vi "State Lua Garbage Collect.vi"(4 "stepmul (majormul)":i32, 6 "stepsize (minormul)":i32, 8 "pause?":bool, 9 "LUA_GC (LUA_GCCOLLECT)":T1=enum."LUA_GCCOLLECT", 10 "error in (no error)":errorcluster, 11 "Lua in":refnum<class "Lua.lvclass">) -> (1 "result":i32, 2 "error out":errorcluster, 3 "Lua out":refnum<class "Lua.lvclass">)   [LabVIEW 2020, in "Lua for LabVIEW.lvlib" / "Lua.lvclass"]
doc: "Controls the garbage collector.\n\nThis function performs several tasks, according to the value of the parameter what. For options that need extra arguments, they are listed after the option.\n\nLUA_GCCOLLECT: Performs a full garbage-collection cycle.\nLUA_GCSTOP: Stops the garbage collector.\nLUA_GCRESTART: Restarts the garbage collector.\nLUA_GCCOUNT: Returns the current amount of memory (in Kbytes) in use by Lua.\nLUA_GCCOUNTB: Returns the remainder of dividing the current amount of bytes of memory in use by Lua by 1024.\nLUA_GCSTEP (int stepsize): Performs an incremental step of garbage collection, corresponding to the allocation of stepsize Kbytes.\nLUA_GCISRUNNING: Returns a boolean that tells whether the collector is running (i.e., not stopped).\nLUA_GCINC (int pause, int stepmul, stepsize): Changes the collector to incremental mode with the given parameters (see §2.5.1). Returns the previous mode (LUA_GCGEN or LUA_GCINC).\nLUA_GCGEN (int minormul, int majormul): Changes the collector to generational mode with the given parameters (see §2.5.2). Returns the previous mode (LUA_GCGEN or LUA_GCINC).\nFor more details about these options, see collectgarbage."
uses:
  Lua.lvclass
  lib/lua.dll/types/LUA_GC.ctl
  Lua.lvclass/Lua.ctl
  lib/lua.dll/lua.dll.lvlib
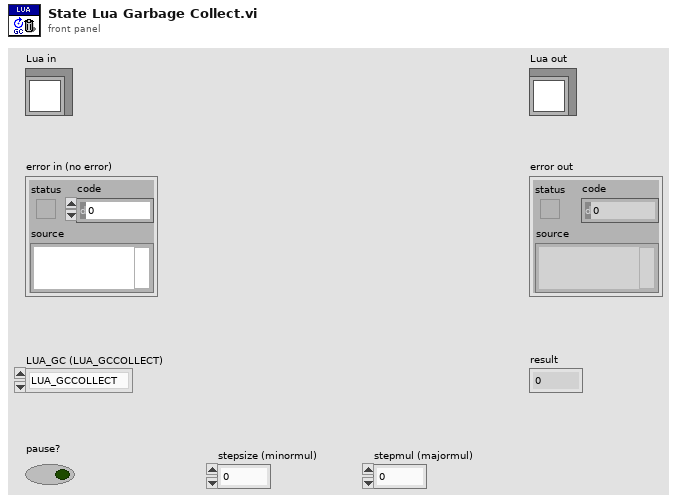
[diagram p1: front panel]
types:
  T1 = typedef "lua.dll.lvlib/LUA_GC.ctl" = enum32{"LUA_GCSTOP", "LUA_GCRESTART", "LUA_GCCOLLECT", "LUA_GCCOUNT", "LUA_GCCOUNTB", "LUA_GCSTEP", "LUA_GCSETPAUSE", "LUA_GCSETSTEPMUL", "LUA_GCSETMAJORINC", "LUA_GCISRUNNING", "LUA_GCGEN", "LUA_GCINC"}
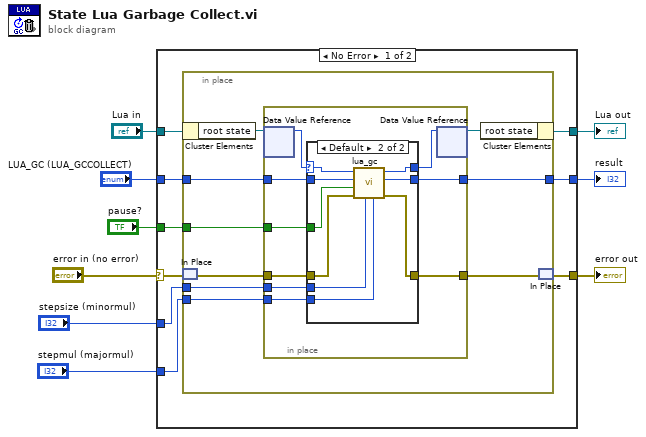
[diagram p0: block diagram]
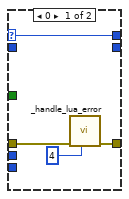
[diagram p2: hidden frame]
diagram:
  n1 = case shown="No Error" "error in (no error)" {
    selector: "error in (no error)" -> [w17 w51]
    tunnel: [w16 w51] -> w8
    tunnel: [w15 w50] -> w6
    tunnel: "Lua in" -> [w18 w50]
    tunnel: "LUA_GC (LUA_GCCOLLECT)" -> [w14 _]
    tunnel: [w13 _] -> w4
    tunnel: "stepmul (majormul)" -> [w12 _]
    tunnel: "stepsize (minormul)" -> [w11 _]
    tunnel: "pause?" -> [w10 _]
    frame No Error {
      n2 = in-place {
        in-place-border: w14 -> [w23]
        in-place-border: [w22] -> w13
        in-place-border: w12 -> [w21]
        in-place-border: w11 -> [w20]
        in-place-border: w10 -> [w19]
        n3 = in-place-cluster #1(w18) -> ("root state"=w25:refnum<data-value>)
        n4 = in-place-match #2(w17) -> (w27:errorcluster)
        n5 = in-place {
          in-place-border: w27 -> [w36]
          in-place-border: [w35] -> w26
          in-place-border: w23 -> [w32]
          in-place-border: [w31] -> w22
          in-place-border: w21 -> [w30]
          in-place-border: w20 -> [w29]
          in-place-border: w19 -> [w28]
          n6 = in-place-dvr #3(w25) -> (w34:u64)  [unwired: 1 out]
          n7 = case shown="Default" w34 {
            selector: w34 -> [w40 w49]
            tunnel: [w40 w48] -> w33
            tunnel: w36 -> [w37 w46]
            tunnel: [w38 w45] -> w35
            tunnel: w32 -> [_ w47]
            tunnel: [_ w44] -> w31
            tunnel: w30 -> [_ w43]
            tunnel: w29 -> [_ w42]
            tunnel: w28 -> [_ w41]
            frame 0 {
              n8 = call "_handle_lua_error.vi"("lua status"=4 ("lua_load errcode"), "error in (no error)"=w37) -> ("error out"=w38:errorcluster)  [unwired: 9 in]
            }
            frame Default {
              n9 = call "lua_gc.vi"("stepmul (majormul)"=w43, "stepsize (minormul)"=w42, "error in (no error)"=w46, "pause?"=w41, "what"=w47, "lua_state_p"=w49) -> ("error out"=w45:errorcluster, "result"=w44:i32, "lua_state_p out"=w48:u64)  [unwired: 3 in]
            }
          }
          n10 = in-place-dvr #3(w33) -> (w24:refnum<data-value>)  [unwired: 1 out]
        }
        n11 = in-place-cluster #1("root state"=w24) -> (w15:refnum<class "Lua.lvclass">)
        n12 = in-place-match #2(w26) -> (w16:errorcluster)
      }
    }
    frame Error {
    }
  }
  "error out" <- w8
  "Lua out" <- w6
  "result" <- w4
